vi "get_value_for_inline_table.vi"(8 "error in (no error)":errorcluster, 11 "Value in":refnum<class "Value.lvclass">) -> (0 "error out":errorcluster, 1 "InlineTable out":refnum<class "InlineTable.lvclass">, 3 "Value out":refnum<class "Value.lvclass">)   [LabVIEW 2020, in "toml_edit.lvlib" / "Value.lvclass"]
uses:
  Value.lvclass
  InlineTable/InlineTable.lvclass
  value_type--enum.ctl
  Value.lvclass/Value.ctl
  dragon_toml_64.dll
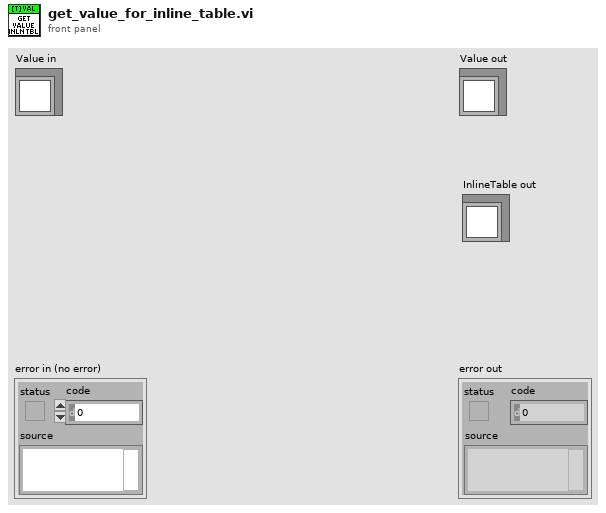
[diagram p1: front panel]
types:
  T1 = typedef "toml_edit.lvlib/Value.lvclass/value_type--enum.ctl" = enum16{"Unknown", "String", "Integer", "Float", "Boolean", "Datetime", "Array", "InlineTable"}
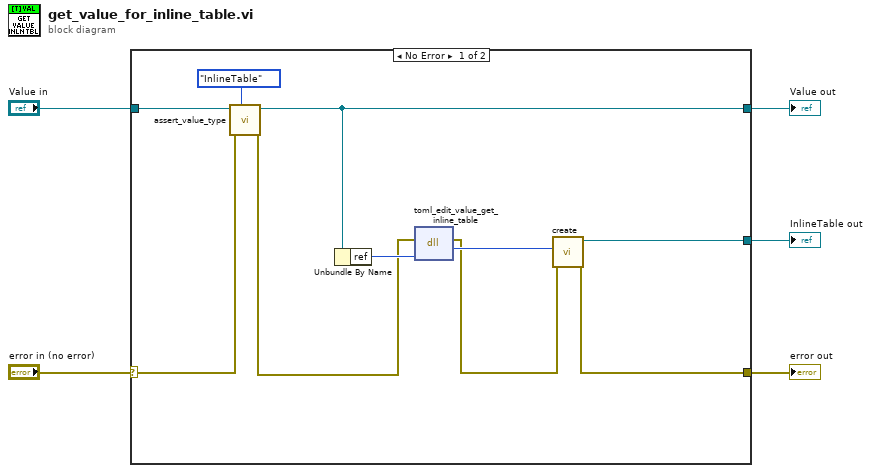
[diagram p0: block diagram]
diagram:
  n1 = case shown="No Error" "error in (no error)" {
    selector: "error in (no error)" -> [w8 w17]
    tunnel: [w12 w17] -> w4
    tunnel: [w10 w16] -> w2
    tunnel: "Value in" -> [w9 w16]
    tunnel: [w13 _] -> w1
    frame No Error {
      n2 = call "assert_value_type.vi"("value_type"=value_type--enum."InlineTable", "error in (no error)"=w8, "Value in"=w9) -> ("error out"=w7:errorcluster, "Value out"=w10:refnum<class "Value.lvclass">)  [unwired: 7 in]
      n3 = Unbundle By Name(w10) -> ("ref"=w15:u64)
      n4 = dll-call lib="C:/Projects/labview-project-load-tools/source/submodules/toml-edit-labview/lv_src/dragon_toml_*.*" fn="toml_edit_value_get_inline_table"(error in=w7, "item_ref"=w15) -> (error out=w11:errorcluster, "table_ptr"=w14:u64)  [unwired: 3 in, 1 out]
      n5 = call "create.vi"("error in (no error)"=w11, "ref"=w14) -> ("error out"=w12:errorcluster, "InlineTable out"=w13:refnum<class "InlineTable.lvclass">)  [unwired: 8 in]
    }
    frame Error {
    }
  }
  "error out" <- w4
  "Value out" <- w2
  "InlineTable out" <- w1
